vi "Extra_Commands_Global.vi"() -> ()   [LabVIEW 2014]
panel:
  in  "Datum Image":string="!Datum Image"
  in  "Add Height to Local Floor Height":string="!Add Height to Local Floor Height"
  out "If command global value":dbl
  in  "!Traverse Setup":string="!Traverse Setup"
  in  "Skip if Sd Error is Below":string="!Skip if Sd Error is Below"
  in  "Minutes Before Repeating Row":string="!Minutes Before Repeating Row"
  in  "Home":string="!Home"
  in  "Pause Until":string="!Pause Until"
  in  "If Command":string="!IF"
  in  "Skip Source Demand":string="!Skip Source Demand"
  in  "Not Using Source":string="!Not Using Source"
  in  "Repeat First Position":string="!Repeat First Position"
  in  "Skip Traverse Position Demand":string="!Skip Traverse Position Demand"
  in  "Establish Exp Conditions (s)":string="!Establish Exp Conditions (s)"
  in  "Skip Tunnel Speed Demand":string="!Skip Tunnel Speed Demand"
  in  "Work in Tunnel Coordinates":string="!Work in Tunnel Coordinates"
  in  "Point Spacing Parameters":string="!Point Spacing Parameters"
  in  "Puff Duration Sec":string="!Puff Duration Sec"
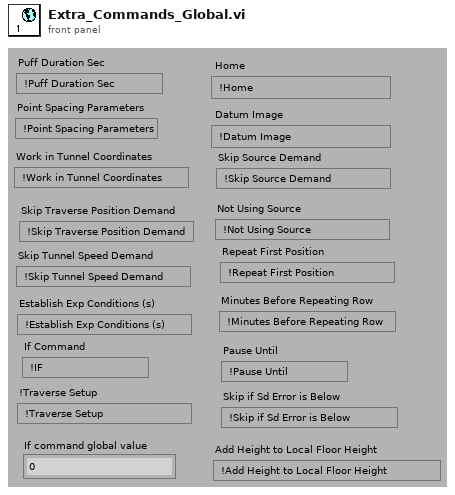
[diagram p1: front panel]
diagram:
